vi "2基礎題-ListBox.vi"() -> ()   [LabVIEW 2019]
panel:
  in  "Stop":bool
  out "商品":string
  out "價格":i32
  in  "品名價格":i32(listbox)=6
  # "1. 以Multicolumn Listbox製作價目表如下；\n2. 程式執行前，先將其中一項的庫存設為無；\n3. 程式執行後，將無庫存的項目Disable；\n4. 點選的項目，會在右邊顯示品名及價格。"
  # "String"
  # "Numeric"
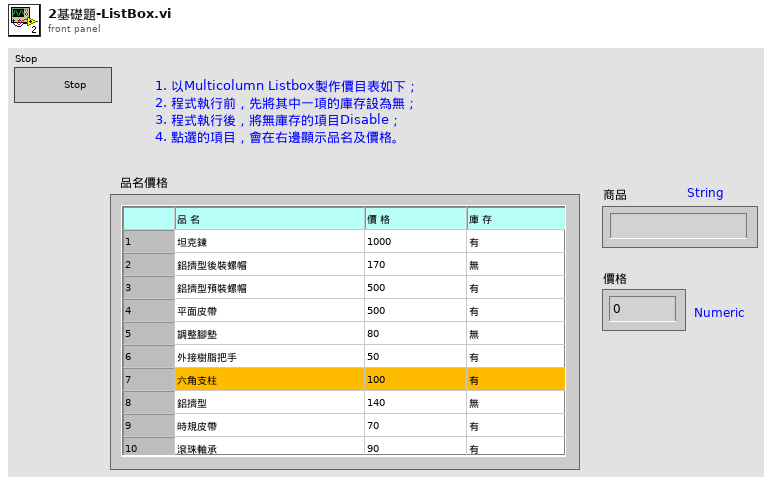
[diagram p1: front panel]
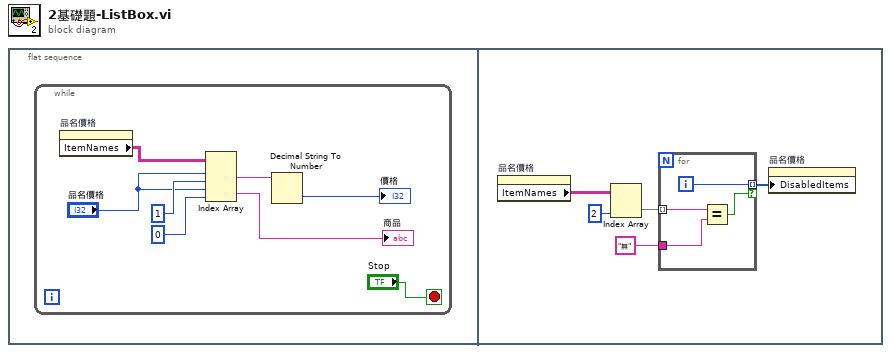
[diagram p0: block diagram]
diagram:
  n1 = flat-sequence {
    frame #0 {
      n2 = while {
        stop <- "Stop" stop-if-true
        n3 = property on="品名價格" class="MCListbox (strict)"() -> ("ItemNames"=w8:string[][])  [unwired: 2 in, 2 out]
        n4 = Index Array(array=w8, index (row) #1="品名價格", index (col) #1=1 ("disabled index (col)"), index (row) #2="品名價格", index (col) #2=0 ("disabled index (col)")) -> (element #1=w6:string, element #2=→"商品":string)
        n5 = Decimal String To Number(string=w6) -> (number=→"價格":i32)  [unwired: 2 in, 1 out]
      }
    }
    frame #1 {
      n6 = property on="品名價格" class="MCListbox (strict)"() -> ("ItemNames"=w11:string[][])  [unwired: 2 in, 2 out]
      n7 = Index Array(array=w11, index (col)=2 ("disabled index (col)")) -> (element=w12:string[])  [unwired: 1 in]
      n8 = for {
        tunnel: w12 -> [w17] mode=indexing
        tunnel: "無" ("y") -> [w16]
        tunnel: [w15] -> w13 mode=indexing if=w14
        i -> [w15]
        n9 = Equal?(x=w17, y=w16) -> (x = y?=w14:bool)
      }
      n10 = property on="品名價格" class="MCListbox (strict)"("DisabledItems"=w13) -> ()  [unwired: 2 in, 2 out]
    }
  }
